vi "SrReplaceStringParser.vi"(8 "error in":errorcluster, 11 "ReplaceString":string) -> (0 "error out":errorcluster, 1 "ReplSubStrNum":i32[](array[numeric]), 2 "ReplStrLengths":i32[](array[numeric]), 3 "ReplStrOffsets":i32[](array[numeric]))   [LabVIEW 2021, in "libpcre2-8.lvlib"]
uses:
  libpcre2-8.lvlib
  Pcre2GetOvectorPointer8.vi
  Pcre2CompileError.vi
  Pcre2FnkCallError.vi
  Pcre2ErrorNull.vi
  Pcre2LibError.vi
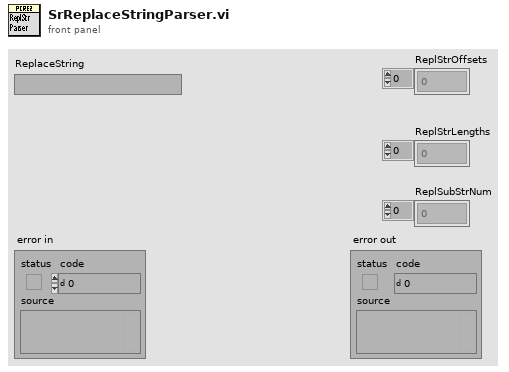
[diagram p1: front panel]
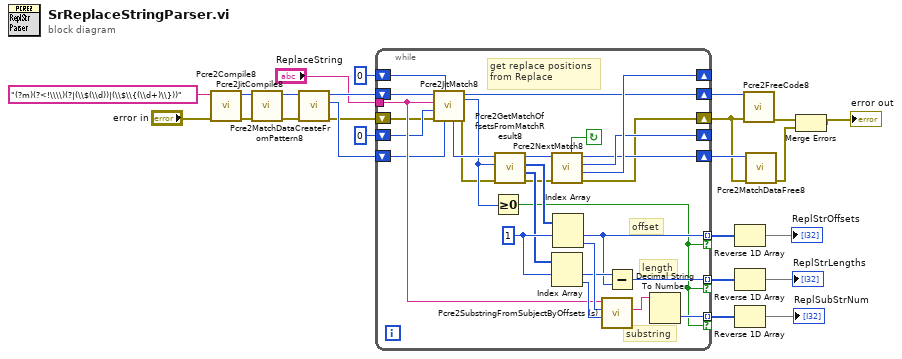
[diagram p0: block diagram]
diagram:
  n1 = call "Pcre2Compile8.vi"("error in"="error in", "Pattern"="(?m)(?<!\\\\)(?|(\\$(\\d))|(\\$\\{(\\d+)\\}))" ("search pattern")) -> ("error out"=w21:errorcluster, "pCode"=w22:u64)  [unwired: 8 in]
  n2 = call "Pcre2JitCompile8.vi"("error in"=w21, "pCode"=w22) -> ("error out"=w18:errorcluster, "pCode"=w20:u64)  [unwired: 8 in]
  n3 = call "Pcre2MatchDataCreateFromPattern8.vi"("error in"=w18, "pCode"=w20) -> ("error out"=w14:errorcluster, "pMatchData"=w17:u64, "pCode"=w19:u64)  [unwired: 7 in]
  n4 = while {
    tunnel: "ReplaceString" -> [w44]
    shift-right: [w35] -> _
    shift-left: u64 0 -> [w43]
    tunnel: [w49] -> w13 mode=indexing if=w31
    tunnel: [w47] -> w12 mode=indexing if=w31
    tunnel: [w46] -> w11 mode=indexing if=w31
    shift-right: [w33] -> w15
    shift-left: w17 -> [w42]
    shift-right: [w36] -> _
    shift-left: u32 0 ("GlobalOptions") -> [w37]
    shift-right: [w34] -> w16
    shift-left: w19 -> [w45]
    shift-right: [w29] -> w10
    shift-left: w14 -> [w30]
    stop <- w26 continue-if-true
    w52 = 1 ("index")
    # "get replace positions\nfrom Replace"
    # "offset"
    # "length"
    # "substring"
    n5 = call "Pcre2JitMatch8.vi"("pMatchData"=w42, "Options"=w37, "error in"=w30, "StartOffset"=w43, "Subject"=w44, "pCode"=w45) -> ("error out"=w28:errorcluster, "MatchResult"=w32:i32, "pCode"=w34:u64, "pMatchData"=w41:u64)  [unwired: 2 in]
    n6 = Greater Or Equal To 0?(x=w32) -> (x >= 0?=w31:bool)
    n7 = call "Pcre2GetMatchOffsetsFromMatchResult8.vi"("error in"=w28, "MatchResult"=w32, "pMatchData"=w41) -> ("error out"=w27:errorcluster, "OffsetsPastMatch"=w40:i32[], "MatchOffsets"=w39:i32[], "pMatchData"=w38:u64)  [unwired: 5 in]
    n8 = call "Pcre2NextMatch8.vi"("error in"=w27, "pMatchData"=w38) -> ("error out"=w29:errorcluster, "GlobalOptions"=w36:u32, "NextStartOffset"=w35:u64, "pMatchData"=w33:u64, "ContinueMatch?"=w26:bool)  [unwired: 5 in]
    n9 = Index Array(array=w40, index #1=w52) -> (element #1=w48:i32, element #2=w50:i32)  [unwired: 1 in]
    n10 = Index Array(array=w39, index #1=w52) -> (element #1=w47:i32, element #2=w51:i32)  [unwired: 1 in]
    n11 = call "Pcre2SubstringFromSubjectByOffsets (s).vi"("OffsetPastMatch"=w50, "MatchOffset"=w51, "Subject"=w44) -> ("Substring"=w25:string)  [unwired: 8 in]
    n12 = Subtract(x=w48, y=w47) -> (x-y=w46:i32)
    n13 = Decimal String To Number(string=w25) -> (number=w49:i32)  [unwired: 2 in, 1 out]
  }
  n14 = Reverse 1D Array(array=w12) -> (reversed array=→"ReplStrOffsets":i32[])
  n15 = Reverse 1D Array(array=w11) -> (reversed array=→"ReplStrLengths":i32[])
  n16 = Reverse 1D Array(array=w13) -> (reversed array=→"ReplSubStrNum":i32[])
  n17 = call "Pcre2FreeCode8.vi"("error in"=w10, "pCode"=w16) -> ("error out"=w3:errorcluster)  [unwired: 9 in]
  n18 = call "Pcre2MatchDataFree8.vi"("error in"=w10, "pMatchData"=w15) -> ("error out"=w2:errorcluster)  [unwired: 9 in]
  n19 = Merge Errors(w3, w2) -> (→"error out":errorcluster)
